vi "Calibrate_Open_One_Freq-OLD.vi"() -> ()   [LabVIEW 2020]
panel:
  out "serial poll byte":i16
  out "error out":errorcluster
  in  "Cal_Delay_Step":u16
  in  "error in":errorcluster
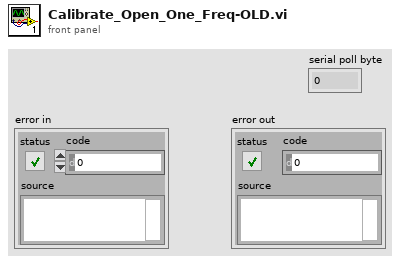
[diagram p1: front panel]
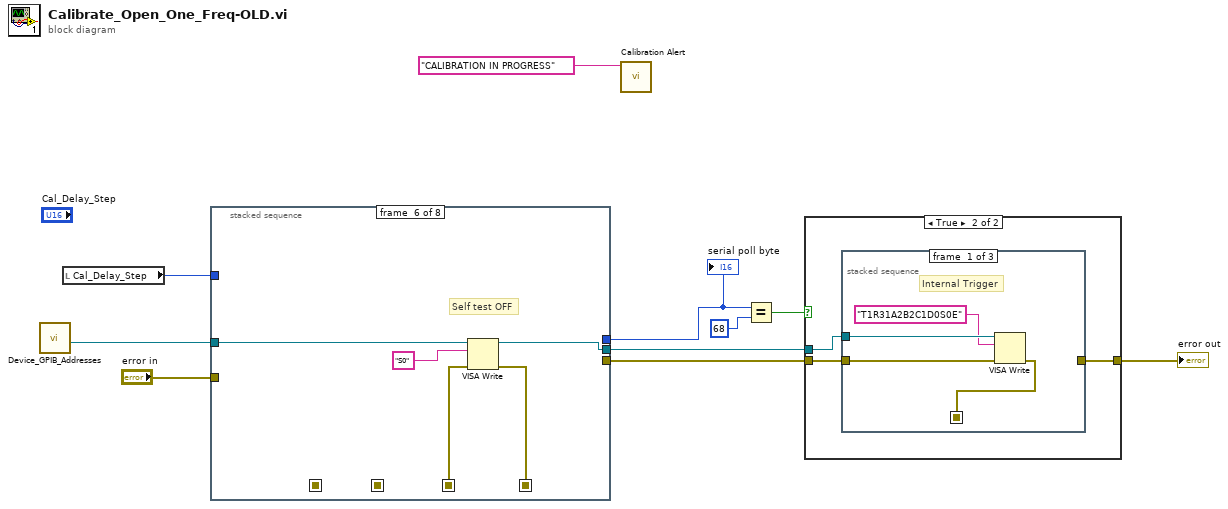
[diagram p0: block diagram]
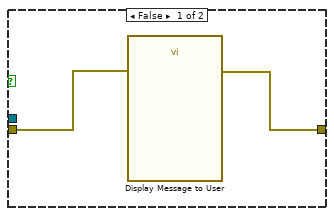
[diagram p2: hidden frame]
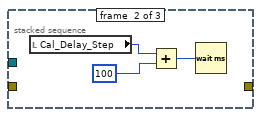
[diagram p3: hidden frame]
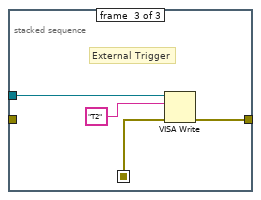
[diagram p4: hidden frame]
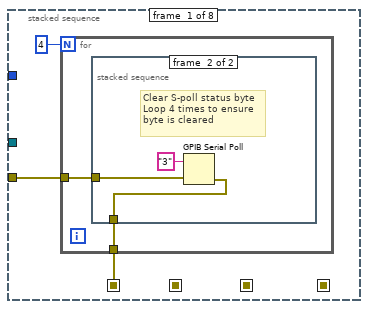
[diagram p5: hidden frame]
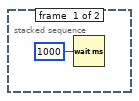
[diagram p6: hidden frame]
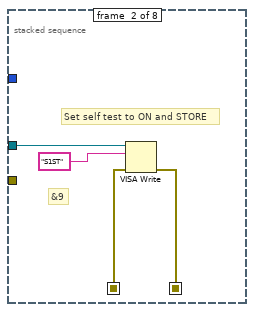
[diagram p7: hidden frame]
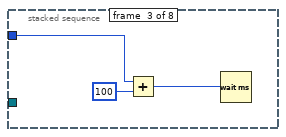
[diagram p8: hidden frame]
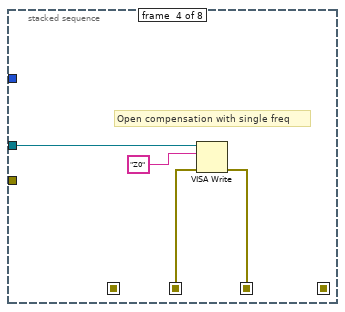
[diagram p9: hidden frame]
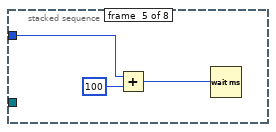
[diagram p10: hidden frame]
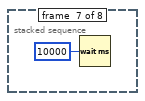
[diagram p11: hidden frame]
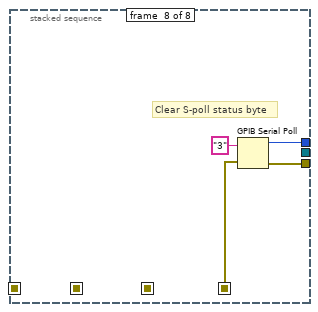
[diagram p12: hidden frame]
diagram:
  n1 = call "Device_GPIB_Addresses.vi"() -> ("HP 4275A Address"=w2:refnum<visa-resource-name>)  [unwired: 9 in, 2 out]
  n2 = local read "Cal_Delay_Step"() -> (w5:u16)
  n3 = stacked-sequence {
    seq-local: [w11 _ _ _ _ _ _ _] -> [_ w21 _ _ _ _ _ _]
    seq-local: [_ w20 _ _ _ _ _ _] -> [_ _ _ w28 _ _ _ _]
    seq-local: [_ _ _ w27 _ _ _ _] -> [_ _ _ _ _ w36 _ _]
    seq-local: [_ _ _ _ _ w35 _ _] -> [_ _ _ _ _ _ _ w43]
    tunnel: "error in" -> [w12 _ _ _ _ _ _ _]
    tunnel: w5 -> [_ _ w26 _ w31 _ _ _]
    tunnel: [_ _ _ _ _ _ _ w42] -> w6
    tunnel: [_ _ _ _ _ _ _ w41] -> w8
    tunnel: w2 -> [_ w23 _ w30 _ w37 _ _]
    tunnel: [_ _ _ _ _ w34 _ _] -> w1
    frame #0 {
      n4 = for {
        N: 4 -> [_]
        tunnel: w12 -> [w15]
        tunnel: [w14] -> w11
        n5 = stacked-sequence {
          tunnel: w15 -> [_ w19]
          tunnel: [_ w18] -> w14
          frame #0 {
            n6 = Wait (ms)(milliseconds to wait=u32 1000) -> ()  [unwired: 1 out]
          }
          frame #1 {
            # "Clear S-poll status byte\nLoop 4 times to ensure\nbyte is cleared"
            n7 = GPIB Serial Poll(0:"3" ("address string"), 1:w19) -> (4:w18:errorcluster)  [unwired: 2 out]
          }
        }
      }
    }
    frame #1 {
      # "&9"
      # "Set self test to ON and STORE"
      n8 = VISA Write(VISA resource name=w23, write buffer="S1ST" ("data"), error in (no error)=w21) -> (error out=w20:errorcluster)  [unwired: 2 out]
    }
    frame #2 {
      n9 = Add(x=w26, y=u16 100) -> (x+y=w24:u16)
      n10 = Wait (ms)(milliseconds to wait=w24) -> ()  [unwired: 1 out]
    }
    frame #3 {
      # "Open compensation with single freq"
      n11 = VISA Write(VISA resource name=w30, write buffer="Z0" ("data"), error in (no error)=w28) -> (error out=w27:errorcluster)  [unwired: 2 out]
    }
    frame #4 {
      n12 = Add(x=w31, y=u16 100) -> (x+y=w32:u16)
      n13 = Wait (ms)(milliseconds to wait=w32) -> ()  [unwired: 1 out]
    }
    frame #5 {
      # "Self test OFF"
      n14 = VISA Write(VISA resource name=w37, write buffer="S0" ("data"), error in (no error)=w36) -> (VISA resource name out=w34:refnum<visa-resource-name>, error out=w35:errorcluster)  [unwired: 1 out]
    }
    frame #6 {
      n15 = Wait (ms)(milliseconds to wait=u32 10000) -> ()  [unwired: 1 out]
    }
    frame #7 {
      # "Clear S-poll status byte"
      n16 = GPIB Serial Poll(0:"3" ("address string"), 1:w43) -> (2:w41:i16, 4:w42:errorcluster)  [unwired: 1 out]
    }
  }
  "serial poll byte" <- w8
  n17 = call "Calibration Alert.vi"("message"="CALIBRATION IN PROGRESS" ("format string")) -> ()  [unwired: 10 in, 1 out]
  n18 = Equal?(x=w8, y=i16 68) -> (x = y?=w9:bool)
  n19 = case shown="True" w9 {
    tunnel: w6 -> [w45 w48]
    tunnel: [w44 w47] -> w4
    tunnel: w1 -> [_ w46]
    frame False {
      n20 = call "Display Message to User"("error in (no error)"=w45) -> ("error out"=w44:errorcluster)  [unwired: 9 in, 1 out]
    }
    frame True {
      n21 = stacked-sequence {
        seq-local: [w50 _ _] -> [_ _ w59]
        tunnel: w48 -> [w49 _ _]
        tunnel: [_ _ w56] -> w47
        tunnel: w46 -> [w52 _ w57]
        frame #0 {
          # "Internal Trigger"
          n22 = VISA Write(VISA resource name=w52, write buffer="T1R31A2B2C1D0S0E" ("Keystate"), error in (no error)=w49) -> (error out=w50:errorcluster)  [unwired: 2 out]
        }
        frame #1 {
          n23 = local read "Cal_Delay_Step"() -> (w55:u16)
          n24 = Add(x=w55, y=u16 100) -> (x+y=w53:u16)
          n25 = Wait (ms)(milliseconds to wait=w53) -> ()  [unwired: 1 out]
        }
        frame #2 {
          # "External Trigger"
          n26 = VISA Write(VISA resource name=w57, write buffer="T2" ("data"), error in (no error)=w59) -> (error out=w56:errorcluster)  [unwired: 2 out]
        }
      }
    }
  }
  "error out" <- w4
